vi "pickering_init_test.vi"() -> ()   [LabVIEW 2020]
uses:
  Realization/PIPX40 Matrix/PIPX40 Matrix.lvclass
panel:
  out "infos":variant[](array[variant])
  out "error out":errorcluster
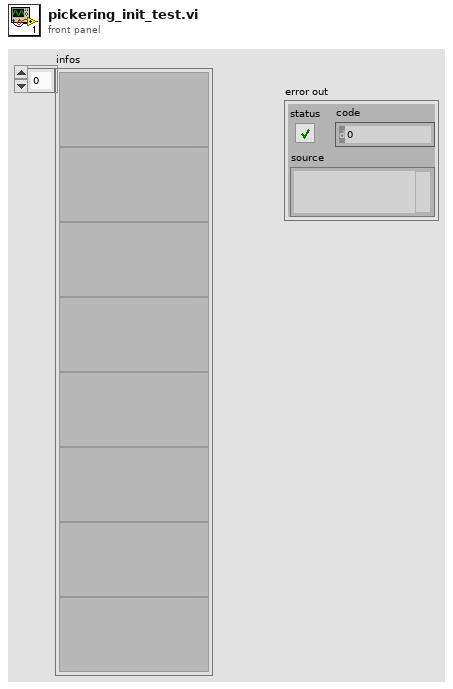
[diagram p1: front panel]
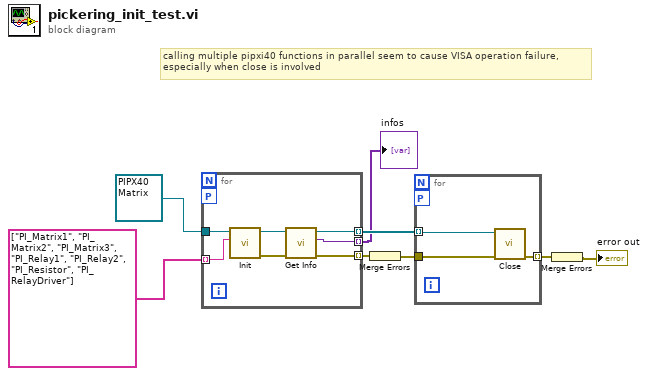
[diagram p0: block diagram]
diagram:
  # "calling multiple pipxi40 functions in parallel seem to cause VISA operation failure,\nespecially when close is involved"
  n1 = for {
    tunnel: string[] ["PI_Matrix1", "PI_Matrix2", "PI_Matrix3", "PI_Relay1", "PI_Relay2", "PI_Resistor", "PI_RelayDriver"] -> [w15] mode=indexing
    tunnel: refnum<class "PIPX40 Matrix.lvclass"> refnum ("PIPXI40 Matrix in") -> [w14]
    workers-P: _ -> [_]
    tunnel: [w11] -> w5 mode=indexing
    tunnel: [w10] -> w3 mode=indexing
    tunnel: [w9] -> w1 mode=indexing
    n2 = call-dynamic "Init.vi"("Params"=w15, "PIPXI40 Base in"=w14) -> ("error out"=w13:errorcluster, "PIPXI40 Base out"=w12:refnum<class "PIPX40 Matrix.lvclass">)  [unwired: 8 in]
    n3 = call-dynamic "Get Info.vi"("error in (no error)"=w13, "PIPXI40 Base in"=w12) -> ("error out"=w11:errorcluster, "Info"=w9:variant, "PIPXI40 Base out"=w10:refnum<class "PIPX40 Matrix.lvclass">)  [unwired: 7 in]
  }
  "infos" <- w1
  n4 = Merge Errors(w5) -> (w4:errorcluster)
  n5 = for {
    tunnel: w4 -> [w17]
    tunnel: w3 -> [w16] mode=indexing
    tunnel: [w18] -> w2 mode=indexing
    workers-P: _ -> [_]
    n6 = call-dynamic "Close.vi"("error in (no error)"=w17, "PIPXI40 Base in"=w16) -> ("error out"=w18:errorcluster)  [unwired: 8 in, 1 out]
  }
  n7 = Merge Errors(w2) -> (→"error out":errorcluster)
